vi "Letter to number.vi"(11 "String":string) -> (2 "T-controller reading type":T1, 3 "Number":i32)   [LabVIEW 2019]
uses:
  Instruments/Temperature Controller/Controls/T-controller reading type.ctl
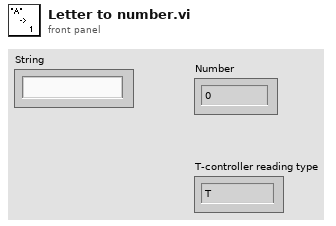
[diagram p1: front panel]
types:
  T1 = typedef "T-controller reading type.ctl" = enum16{"T", "R", "H"}
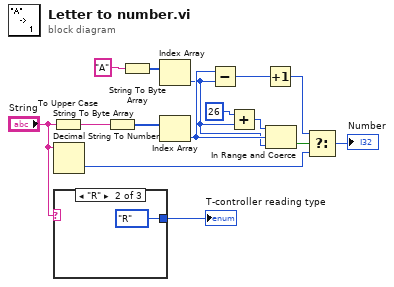
[diagram p0: block diagram]
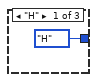
[diagram p2: hidden frame]
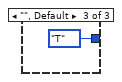
[diagram p3: hidden frame]
diagram:
  n1 = To Upper Case(1:"String") -> (0:w15:string)
  n2 = Decimal String To Number(string="String") -> (number=w8:i32)  [unwired: 2 in, 1 out]
  n3 = case shown="\"R\"" "String" {
    tunnel: [T-controller_reading_type."H" ("T-controller reading type") T-controller_reading_type."R" ("T-controller reading type") T-controller_reading_type."T" ("T-controller reading type")] -> w1
    frame "H" {
    }
    frame "R" {
    }
    frame "", Default {
    }
  }
  "T-controller reading type" <- w1
  n4 = String To Byte Array(string=w15) -> (unsigned byte array=w14:u8[])
  n5 = String To Byte Array(string="A") -> (unsigned byte array=w13:u8[])
  n6 = Index Array(array=w13) -> (element=w4:u8)  [unwired: 1 in]
  n7 = Index Array(array=w14) -> (element=w5:u8)  [unwired: 1 in]
  n8 = Subtract(x=w5, y=w4) -> (x-y=w6:u8)
  n9 = Add(x=u8 26, y=w4) -> (x+y=w10:u8)
  n10 = Increment(x=w6) -> (x+1=w3:u8)
  n11 = In Range and Coerce(upper limit=w10, x=w5, lower limit=w4) -> (In Range?=w9:bool)  [unwired: 1 out]
  n12 = Select(t=w3, s=w9, f=w8) -> (s? t:f=→"Number":i32)
